vi "CancelPurchase.vi"(8 "error in (no error)":errorcluster, 11 "Messages Actor in":refnum<class "Messages Actor.lvclass">) -> (0 "error out":errorcluster, 3 "Messages Actor out":refnum<class "Messages Actor.lvclass">)   [LabVIEW 2020, in "Messages Actor.lvlib" / "Messages Actor.lvclass"]
uses:
  Messages Actor.lvclass
  C:/Program Files (x86)/National Instruments/LabVIEW 2020/vi.lib/ActorFramework/Actor/Actor.lvclass
  <vilib>/ActorFramework/Actor/Actor.lvclass/Actor.ctl
  <vilib>/ActorFramework/Message Enqueuer/Message Enqueuer.lvclass/Message Enqueuer.ctl
  Messages Actor.lvclass/Messages Actor.ctl
  Messages Actor Messages/UpdateChange Msg/UpdateChange Msg.lvclass/UpdateChange Msg.ctl
  <vilib>/ActorFramework/Message Enqueuer/Init from Existing Queue.vi
  <vilib>/ActorFramework/Message Enqueuer/Enqueue.vi
  Messages Actor Messages/UpdateChange Msg/UpdateChange Msg.lvclass
  C:/Program Files (x86)/National Instruments/LabVIEW 2020/vi.lib/ActorFramework/Message/Message.lvclass
  Messages Actor Messages/ResetCredit Msg/ResetCredit Msg.lvclass
  <vilib>/ActorFramework/Message Priority Queue/Priority Enqueue.vi
  <vilib>/ActorFramework/Message Enqueuer/Message Enqueuer.lvclass
  <vilib>/ActorFramework/Actor/Actor.lvclass
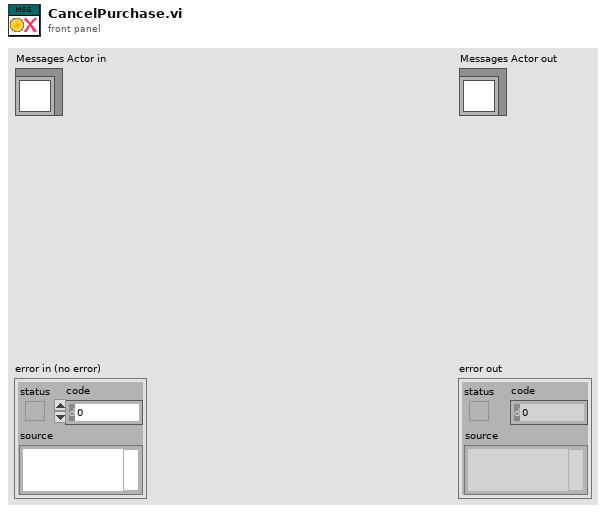
[diagram p1: front panel]
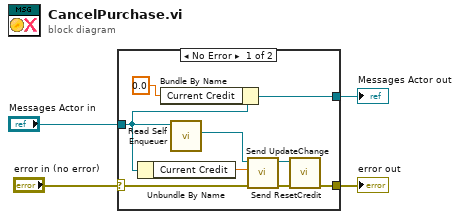
[diagram p0: block diagram]
diagram:
  n1 = case shown="No Error" "error in (no error)" {
    selector: "error in (no error)" -> [w12 w15]
    tunnel: [w10 w15] -> w3
    tunnel: [w6 w14] -> w1
    tunnel: "Messages Actor in" -> [w13 w14]
    frame No Error {
      n2 = Unbundle By Name(w13) -> ("Current Credit"=w7:dbl)
      n3 = Bundle By Name(cluster=w13, "Current Credit"=0.0) -> (w6:refnum<class "Messages Actor.lvclass">)
      n4 = call <vilib>:"Read Self Enqueuer.vi"("Actor"=w13) -> ("Self Enqueuer"=w8:refnum<class "Message Enqueuer.lvclass">)  [unwired: 10 in]
      n5 = call "Send UpdateChange.vi"("error in (no error)"=w12, "Change"=w7, "Message Enqueuer"=w8) -> ("error out"=w11:errorcluster, "Message Enqueuer out"=w9:refnum<class "Message Enqueuer.lvclass">)  [unwired: 7 in]
      n6 = call "Send ResetCredit.vi"("error in (no error)"=w11, "Message Enqueuer"=w9) -> ("error out"=w10:errorcluster)  [unwired: 8 in, 1 out]
    }
    frame Error {
    }
  }
  "error out" <- w3
  "Messages Actor out" <- w1
